vi "flir_dll_test.vi"() -> ()   [LabVIEW 2013]
uses:
  <vilib>/Utility/miscctls.llb/LVRangeTypeDef.ctl
  <userlib>/test_win32dll_d/test_win32dll_d.lvlib
panel:
  in  "IPadderss":string="169.254.96.112"
  out "최소값":dbl
  out "Z 스케일.범위":T1
  in  "정지":bool
  out "최대값":dbl
  out "강도 그래프":dbl[][](graph)
  out "숫자형 3":i32
  in  "Y pixel":i32=160
  in  "X pixel":i32=64
  out "배열":dbl[][](array[numeric])
  out "function return 7":i32
  out "temp":dbl
  out "function return 6":i32
  out "function return 4":i32
  out "function return 3":i32
  out "function return 2":i32
  out "function return":i32
  # "128"
  # "160"
  # "320 256"
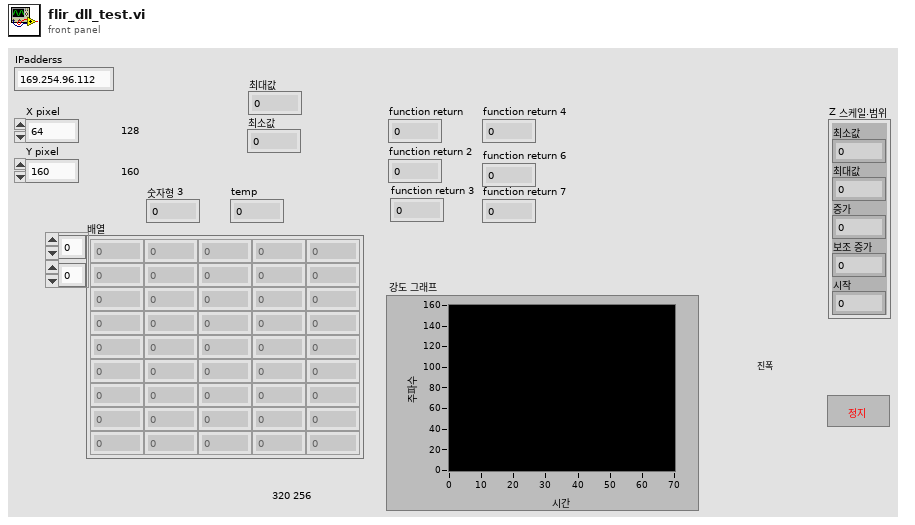
[diagram p1: front panel]
types:
  T1 = typedef "LVRangeTypeDef.ctl" = cluster{"Minimum":dbl, "Maximum":dbl, "Increment":dbl, "Minor Increment":dbl, "Start":dbl}
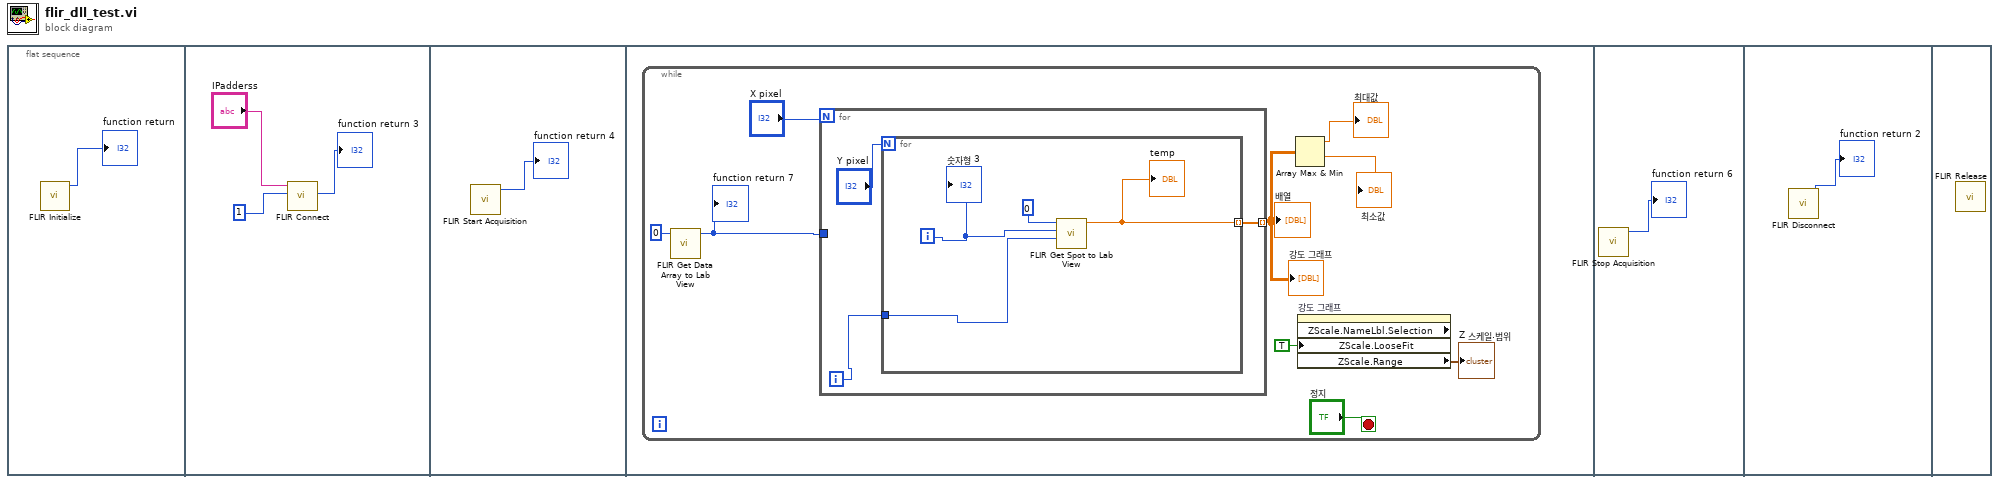
[diagram p0: block diagram]
diagram:
  n1 = flat-sequence {
    frame #0 {
      n2 = call <userlib>:"FLIR Initialize.vi"() -> ("function return"=→"function return":i32)  [unwired: 11 in]
    }
    frame #1 {
      n3 = call <userlib>:"FLIR Connect.vi"("nValue"=1, "IPadderss"="IPadderss") -> ("function return"=→"function return 3":i32)  [unwired: 8 in, 1 out]
    }
    frame #2 {
      n4 = call <userlib>:"FLIR Start Acquisition.vi"() -> ("function return"=→"function return 4":i32)  [unwired: 11 in]
    }
    frame #3 {
      n5 = while {
        stop <- "정지" stop-if-true
        n6 = call <userlib>:"FLIR Get Data Array to Lab View.vi"("nFormat"=0) -> ("function return"=w10:i32)  [unwired: 10 in]
        "function return 7" <- w10
        n7 = for {
          N: "X pixel" -> [_]
          tunnel: [w15] -> w13 mode=indexing
          tunnel: w10 -> [_]
          i -> [w16]
          n8 = for {
            N: "Y pixel" -> [_]
            tunnel: w16 -> [w19]
            tunnel: [w18] -> w15 mode=indexing
            i -> [w20]
            n9 = call <userlib>:"FLIR Get Spot to Lab View.vi"("nYposition"=w19, "nXposition"=w20, "nTemperatureType"=0) -> ("function return"=w18:dbl)  [unwired: 8 in]
            "temp" <- w18
            "숫자형 3" <- w20
          }
        }
        "배열" <- w13
        "강도 그래프" <- w13
        n10 = Array Max & Min(array=w13) -> (max value=→"최대값":dbl, min value=→"최소값":dbl)  [unwired: 2 out]
        n11 = property on="강도 그래프" class="IntGraph (엄격한)" props=["ZScale", "NameLbl", "Selection", "ZScale", "LooseFit", "ZScale", "Range"]("ZScale.LooseFit"=TRUE ("Z 스케일.스케일에 맞춤")) -> ("ZScale.Range"=→"Z 스케일.범위":T1)  [unwired: 2 in, 3 out]
      }
    }
    frame #4 {
      n12 = call <userlib>:"FLIR Stop Acquisition.vi"() -> ("function return"=→"function return 6":i32)  [unwired: 11 in]
    }
    frame #5 {
      n13 = call <userlib>:"FLIR Disconnect.vi"() -> ("function return"=→"function return 2":i32)  [unwired: 11 in]
    }
    frame #6 {
      n14 = call <userlib>:"FLIR Release.vi"() -> ()  [unwired: 12 in]
    }
  }
